vi "2.vi"   [LabVIEW 2015]
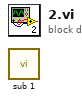
[diagram p0: block diagram]
diagram:
  n1 = call "sub 1.vi"() -> ()  [unwired: 11 in, 1 out]
